vi "Array.vi"() -> ()   [LabVIEW 2021]
panel:
  in  "Length":dbl
  in  "Index":dbl
  in  "Mult":dbl
  out "Sub Array":dbl[](array[numeric]) format="%#.2f"
  out "Array Final":dbl[](array[numeric]) format="%#.2f"
  out "Array":dbl[](array[numeric]) format="%#.2f"
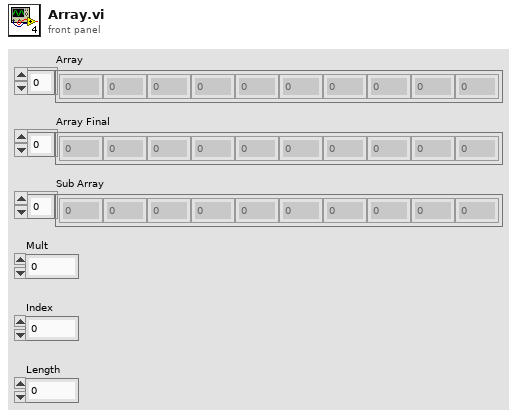
[diagram p1: front panel]
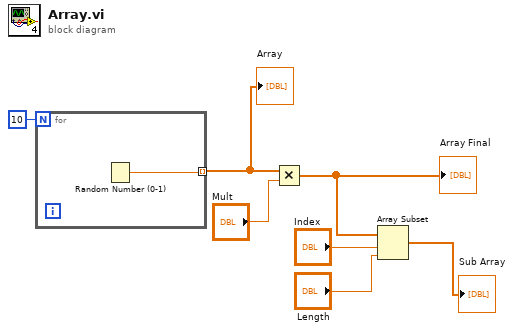
[diagram p0: block diagram]
diagram:
  n1 = for {
    N: 10 -> [_]
    tunnel: [w8] -> w5 mode=indexing
    n2 = Random Number (0-1)() -> (number: 0 to 1=w8:dbl)
  }
  "Array" <- w5
  n3 = Multiply(x=w5, y="Mult") -> (x*y=w3:dbl[])
  "Array Final" <- w3
  n4 = Array Subset(array=w3, index="Index", length="Length") -> (→"Sub Array":dbl[])
